vi "Logging Message Loop_temp.vi"(8 "error in (no error)":errorcluster, 10 "Data Queue":refnum<queue>, 11 "Message Queues":T1) -> (0 "error out":errorcluster)   [LabVIEW 2016]
doc: "The message loop subVI to handle messages pertaining to logging data."
uses:
  support/Message Queue/All Message Queues.ctl
  support/Message Queue/Message Cluster.ctl
  Logging Configuration.ctl
  Logging State.ctl
  support/Message Queue/Enqueue Message (Single).vi
  <vilib>/Utility/error.llb/Error Cluster From Error Code.vi
  <vilib>/ErrorRing/Error Ring.xnode
  Logging.lvlib
  support/Message Queue/Message Queue.lvlib
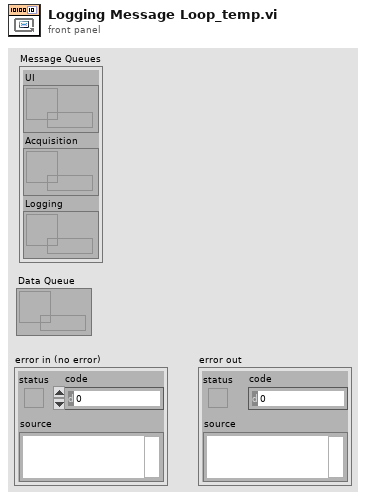
[diagram p1: front panel]
types:
  T1 = typedef "Message Queue.lvlib/All Message Queues.ctl" = cluster{"UI":refnum<queue>, "Acquisition":refnum<queue>, "Logging":refnum<queue>}
  T2 = typedef "Logging.lvlib/Logging State.ctl" = cluster{"State":enum16{"Logging", "Not Logging", "Idle"}, "Samples to Save":u32, "Force Trigger":bool}
  T3 = typedef "Logging.lvlib/Logging Configuration.ctl" = cluster{"Log File Base Path":path, "TDMS File Reference":refnum<k34>, "Samples to Save":u32, "Trigger - Time":u32, "Trigger - Threshold":dbl, "Trigger - Channel":u32, "Enable Time Trigger":bool, "Enable Threshold Trigger":bool, "Always Log":bool}
  T4 = enum16{"open", "open or create", "create or replace", "create", "open (read-only)"}
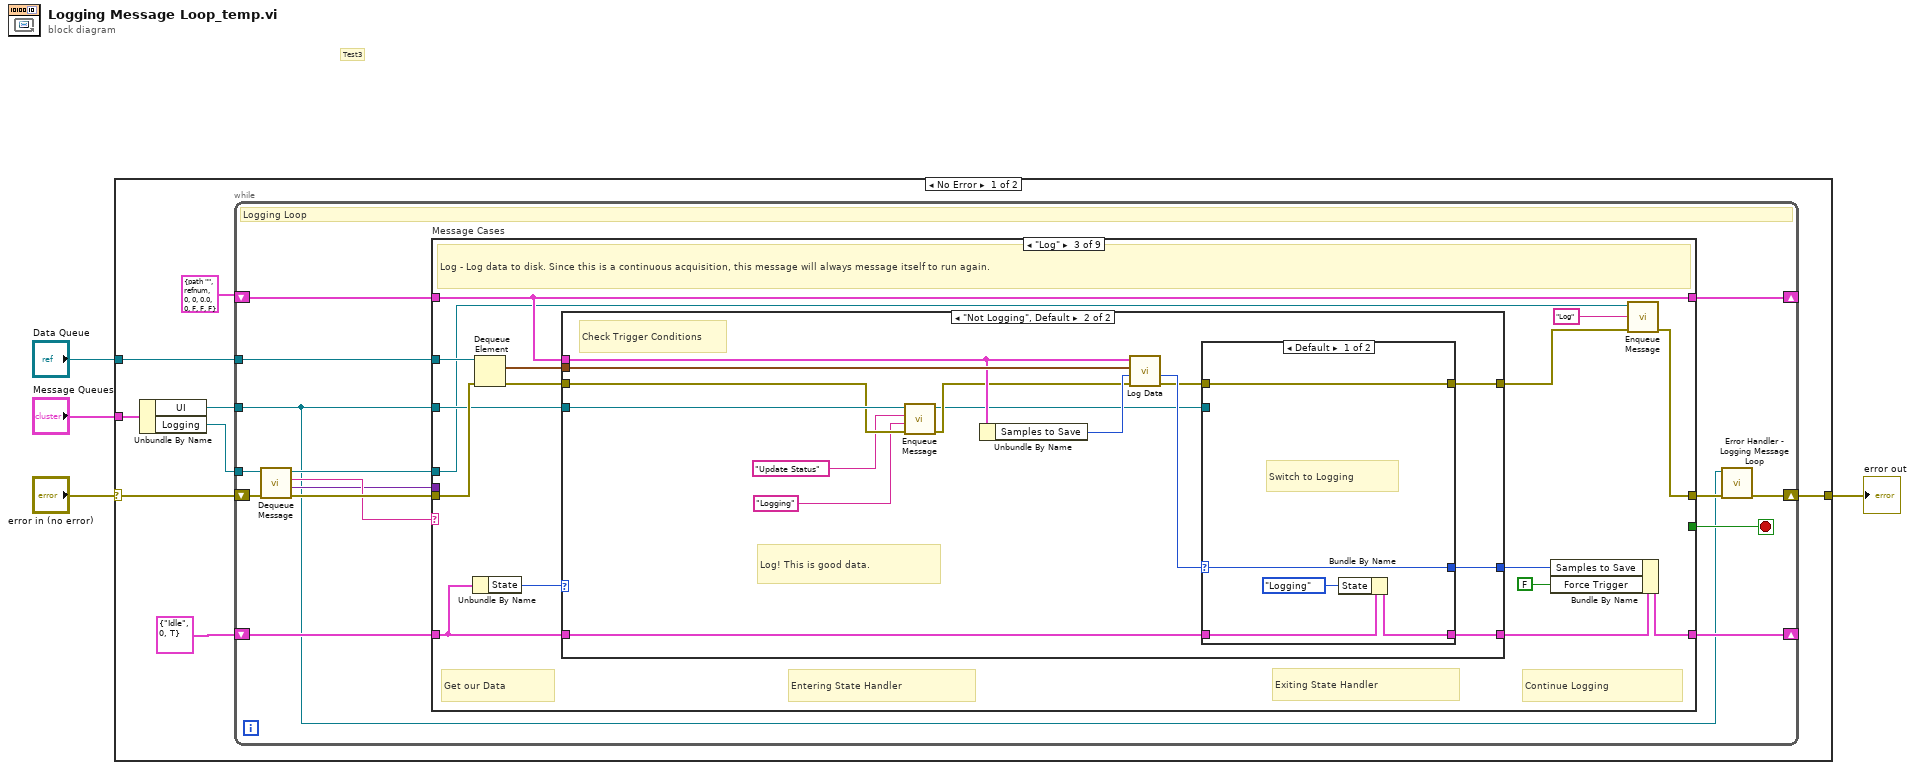
[diagram p0: block diagram]
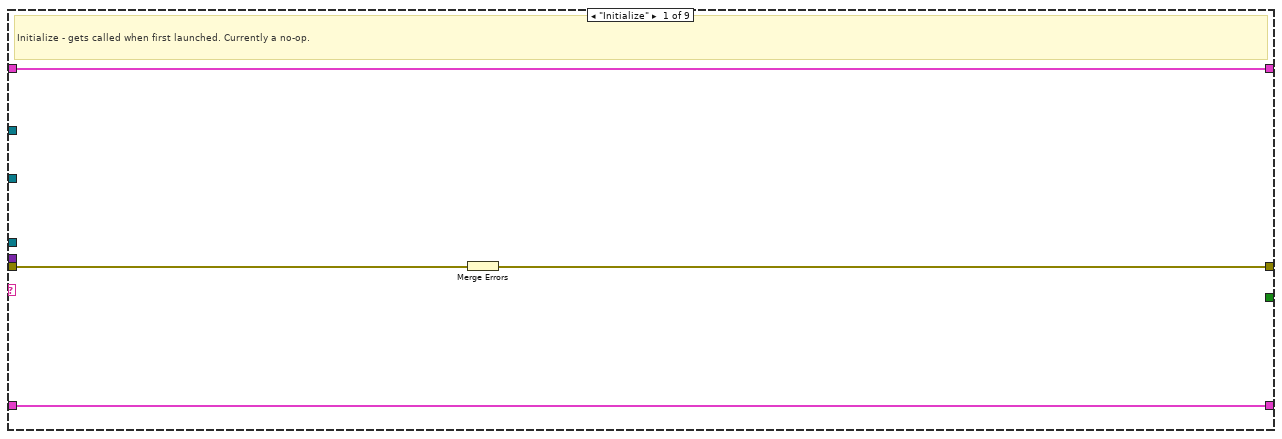
[diagram p2: hidden frame]
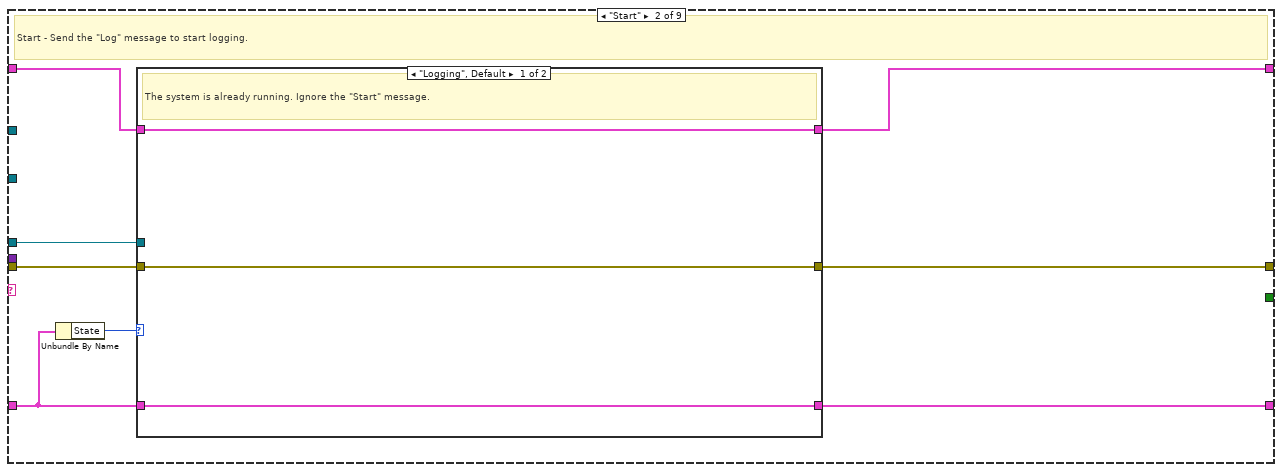
[diagram p3: hidden frame]
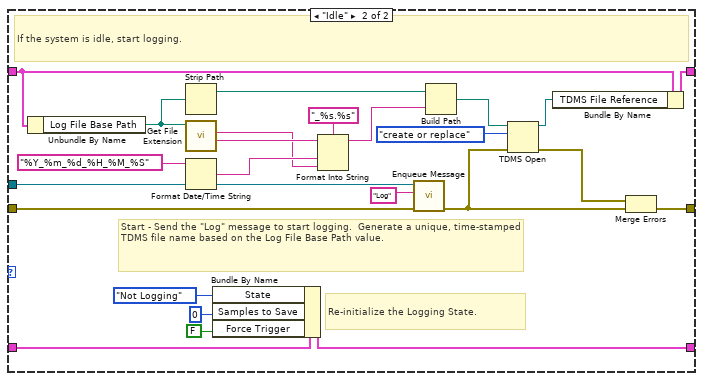
[diagram p4: hidden frame]
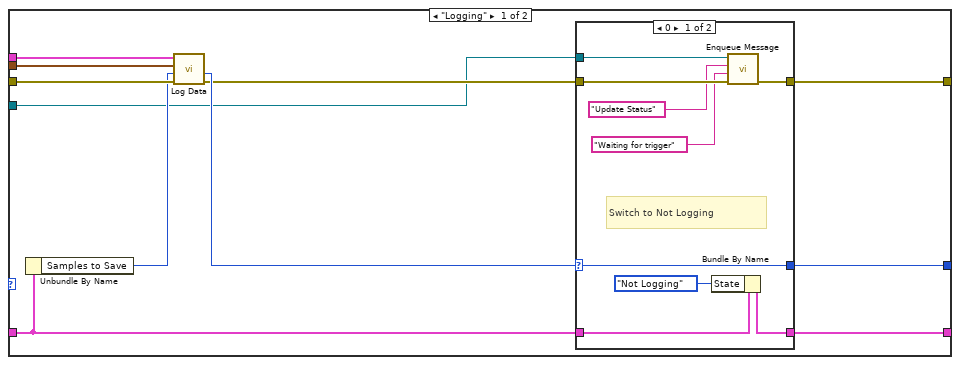
[diagram p5: hidden frame]
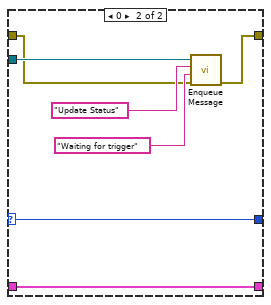
[diagram p7: hidden frame]
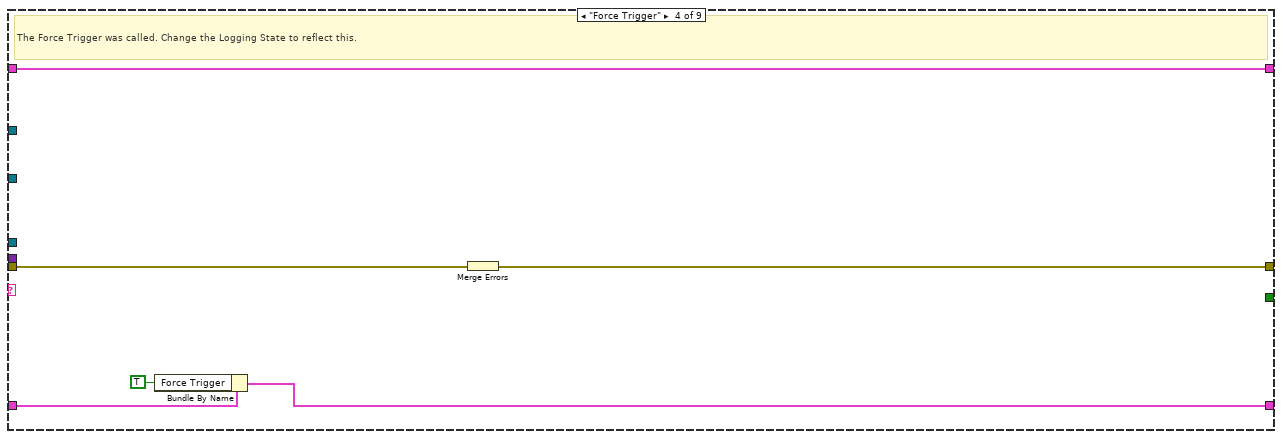
[diagram p8: hidden frame]
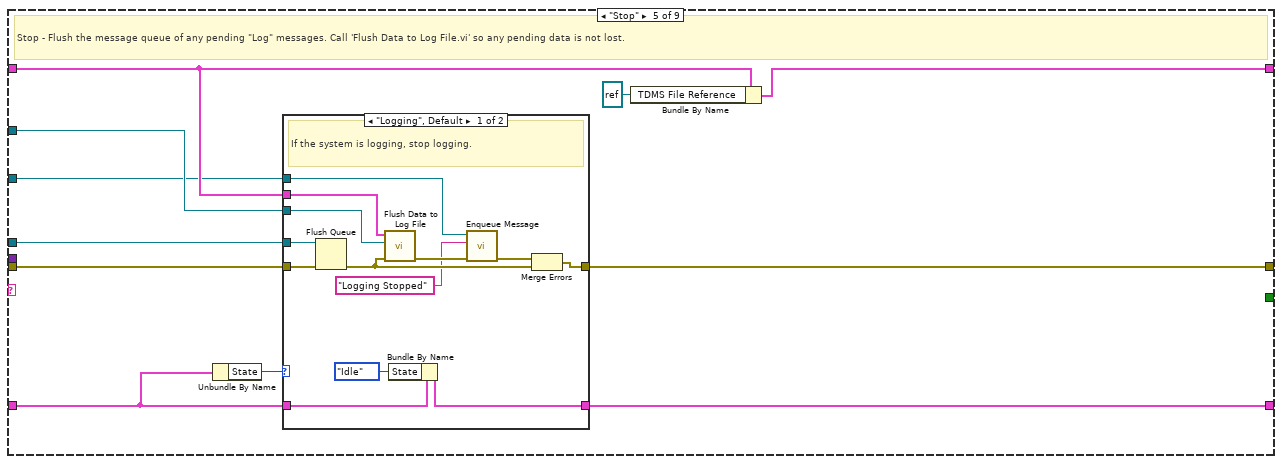
[diagram p9: hidden frame]
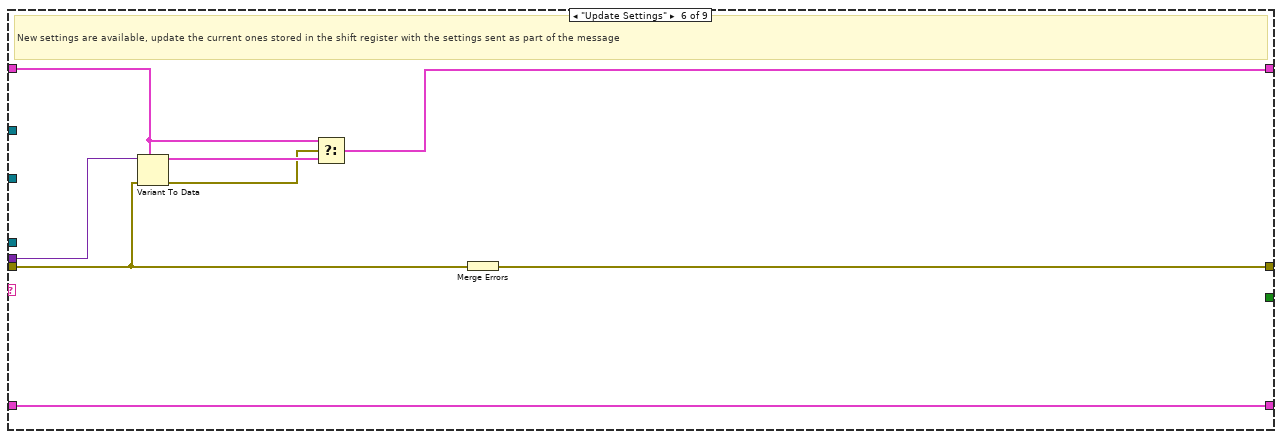
[diagram p11: hidden frame]
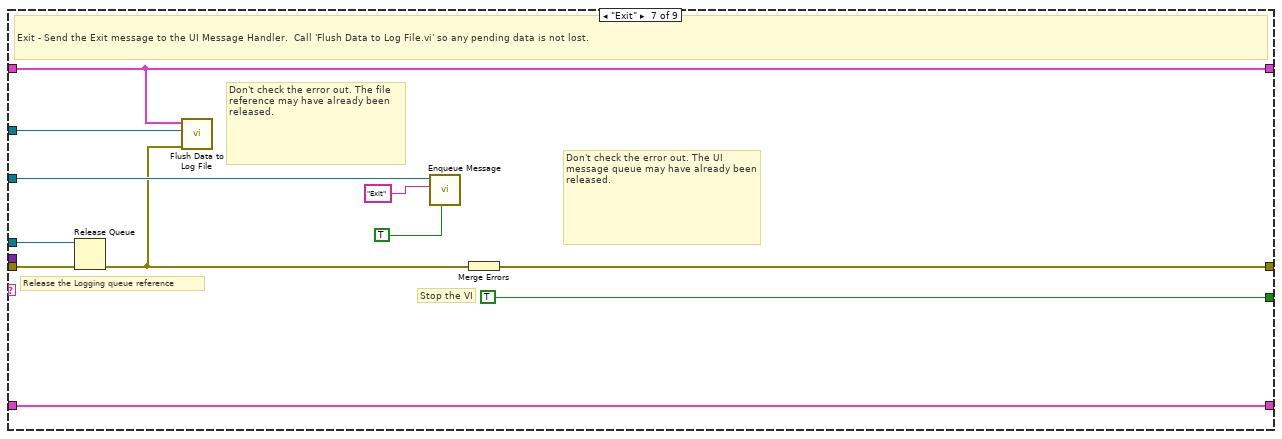
[diagram p12: hidden frame]
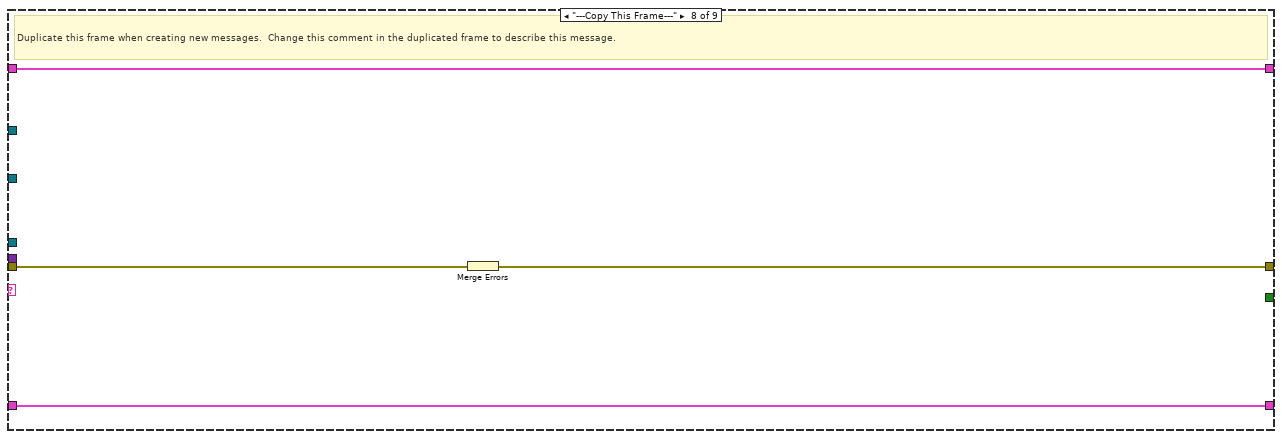
[diagram p13: hidden frame]
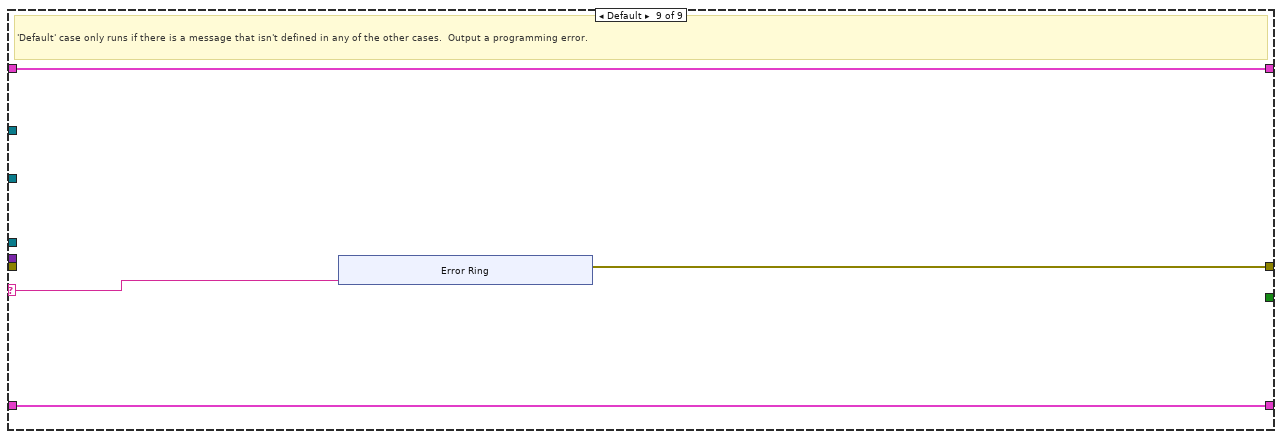
[diagram p14: hidden frame]
diagram:
  # "Test3"
  n1 = case shown="No Error" "error in (no error)" {
    selector: "error in (no error)" -> [w8 w199]
    tunnel: "Message Queues" -> [w12 _]
    tunnel: [w10 w199] -> w3
    tunnel: "Data Queue" -> [w7 _]
    frame No Error {
      n2 = Unbundle By Name(w12) -> ("UI"=w6:refnum<queue>, "Logging"=w11:refnum<queue>)
      n3 = while {
        tunnel: w11 -> [w19]
        shift-right: [w26] -> _
        shift-left: T3 {"Log File Base Path"=path "", "TDMS File Reference"=refnum, "Samples to Save"=0, "Trigger - Time"=0, "Trigger - Threshold"=0.0, "Trigger - Channel"=0, "Enable Time Trigger"=FALSE, "Enable Threshold Trigger"=FALSE, "Always Log"=FALSE} ("Logging Configuration") -> [w27]
        shift-right: [w14] -> w10
        shift-left: w8 -> [w24]
        tunnel: w6 -> [w13]
        tunnel: w7 -> [w18]
        shift-right: [w16] -> _
        shift-left: T2 {"State"=enum."Idle", "Samples to Save"=0, "Force Trigger"=TRUE} -> [w17]
        stop <- w25 stop-if-true
        # "Logging Loop"
        n4 = call "Dequeue Message.vi"("error in (no error)"=w24, "Message Queue"=w19) -> ("error out"=w23:errorcluster, "Message Data"=w21:variant, "Message"=w22:string, "dup Message Queue"=w20:refnum<queue>)  [unwired: 6 in]
        n5 = case "Message Cases" shown="\"Log\"" w22 {
          selector: w22 -> [_ _ _ _ _ _ _ _ w188]
          tunnel: w20 -> [_ w38 w70 _ w147 _ w177 _ _]
          tunnel: w23 -> [w29 w37 w80 w138 w148 w166 w180 w187 _]
          tunnel: [w31 w39 w82 w136 w149 w172 w182 w185 w189] -> w15
          tunnel: w27 -> [w30 w36 w75 w137 w144 w170 w176 w186 w191]
          tunnel: [w30 w35 w75 w137 w146 w167 w176 w186 w191] -> w26
          tunnel: [_ _ _ _ _ _ TRUE _ _] -> w25
          tunnel: w21 -> [_ _ _ _ _ w171 _ _ _]
          tunnel: w13 -> [_ _ w74 _ w142 _ w181 _ _]
          tunnel: w18 -> [_ _ w71 _ w143 _ w175 _ _]
          tunnel: w17 -> [w28 w33 w78 w135 w140 w165 w173 w184 w190]
          tunnel: [w28 w34 w73 w134 w139 w165 w173 w184 w190] -> w16
          frame "Initialize" {
            # "Initialize - gets called when first launched. Currently a no-op."
            n6 = Merge Errors(w29) -> (w31:errorcluster)
          }
          frame "Start" {
            # "Start - Send the \"Log\" message to start logging."
            n7 = Unbundle By Name(w33) -> ("State"=w32:enum16{"Logging", "Not Logging", "Idle"})
            n8 = case shown="\"Logging\", Default" w32 {
              tunnel: [w41 w66] -> w39
              tunnel: w38 -> [_ w65]
              tunnel: w37 -> [w41 w63]
              tunnel: w36 -> [w42 w54]
              tunnel: [w42 w51] -> w35
              tunnel: w33 -> [w40 w47]
              tunnel: [w40 w46] -> w34
              frame "Logging", Default {
                # "The system is already running. Ignore the \"Start\" message."
              }
              frame "Idle" {
                # "Re-initialize the Logging State."
                # "Start - Send the \"Log\" message to start logging.  Generate a unique, time-stamped TDMS file name based on the Log File Base Path value."
                # "If the system is idle, start logging."
                n9 = Unbundle By Name(w54) -> ("Log File Base Path"=w61:path)
                n10 = Strip Path(path=w61) -> (stripped path=w60:path)  [unwired: 1 out]
                n11 = call <vilib>:"Get File Extension.vi"("file"=w61) -> ("filename without extension"=w59:string, "lowercase file extension"=w56:string)  [unwired: 6 in, 3 out]
                n12 = Format Date/Time String(time format string (%c)="%Y_%m_%d_%H_%M_%S") -> (date/time string=w57:string)  [unwired: 2 in]
                n13 = Bundle By Name(cluster=w47, "State"=enum16{"Logging", "Not Logging"}."Not Logging", "Samples to Save"=u32 0 ("Reads to Save"), "Force Trigger"=FALSE) -> (w46:T2)
                n14 = Format Into String(format string="_%s.%s", initial string=w59, w57, w56) -> (resulting string=w55:string)  [unwired: 1 in, 1 out]
                n15 = call-poly "Enqueue Message.vi"("error in (no error)"=w63, "Message"="Log", "Message Queue"=w65) -> ("error out"=w49:errorcluster)  [unwired: 7 in, 1 out]
                n16 = Build Path(base path=w60, name or relative path=w55) -> (appended path=w52:path)
                n17 = TDMS Open(8:w49, 10:T4."create or replace" ("operation (0:open)"), 11:w52) -> (0:w48:errorcluster, 3:w53:refnum<k34>)  [unwired: 4 in]
                n18 = Bundle By Name(cluster=w54, "TDMS File Reference"=w53) -> (w51:T3)
                n19 = Merge Errors(w48, w49) -> (w66:errorcluster)
              }
            }
          }
          frame "Log" {
            # "Exiting State Handler"
            # "Continue Logging"
            # "Entering State Handler"
            # "Get our Data"
            # "Log - Log data to disk. Since this is a continuous acquisition, this message will always message itself to run again."
            n20 = Unbundle By Name(w78) -> ("State"=w79:enum16{"Logging", "Not Logging", "Idle"})
            n21 = Dequeue Element(queue=w71, error in (no error)=w80) -> (element=w77:waveform(dbl)[], error out=w76:errorcluster)  [unwired: 1 in, 2 out]
            n22 = case shown="\"Not Logging\", Default" w79 {
              tunnel: [w87 w120] -> w69
              tunnel: w78 -> [w88 w118]
              tunnel: w77 -> [w92 w114]
              tunnel: w76 -> [w91 w115]
              tunnel: w75 -> [w93 w113]
              tunnel: w74 -> [w83 w117]
              tunnel: [w84 w119] -> w67
              tunnel: [w86 w116] -> w68
              frame "Logging" {
                n23 = Unbundle By Name(w88) -> ("Samples to Save"=w90:u32)
                n24 = call "Log Data.vi"("error in (no error)"=w91, "Samples to Save In"=w90, "Data"=w92, "Logging Configuration"=w93) -> ("error out"=w85:errorcluster, "Samples to Save Out"=w89:u32)  [unwired: 6 in]
                n25 = case shown="0" w89 {
                  selector: w89 -> [w99 w105]
                  tunnel: w85 -> [w97 w104]
                  tunnel: [w98 w104] -> w84
                  tunnel: w88 -> [w101 w103]
                  tunnel: [w100 w103] -> w87
                  tunnel: [w99 w105] -> w86
                  tunnel: w83 -> [w94 _]
                  frame 0 {
                    # "Switch to Not Logging"
                    n26 = Bundle By Name(cluster=w101, "State"=enum16{"Logging", "Not Logging"}."Not Logging") -> (w100:T2)
                    n27 = call-poly "Enqueue Message.vi"("error in (no error)"=w97, "Message Data"="Waiting for trigger" ("Waiting for trigger"), "Message"="Update Status", "Message Queue"=w94) -> ("error out"=w98:errorcluster)  [unwired: 6 in, 1 out]
                  }
                  frame Default {
                    # "Continue in our same State."
                  }
                }
              }
              frame "Not Logging", Default {
                # "Log! This is good data."
                # "Check Trigger Conditions"
                n28 = call-poly "Enqueue Message.vi"("error in (no error)"=w115, "Message Data"="Logging" ("Logging"), "Message"="Update Status", "Message Queue"=w117) -> ("error out"=w109:errorcluster, "dup Message Queue"=w106:refnum<queue>)  [unwired: 6 in]
                n29 = Unbundle By Name(w113) -> ("Samples to Save"=w110:u32)
                n30 = call "Log Data.vi"("error in (no error)"=w109, "Samples to Save In"=w110, "Data"=w114, "Logging Configuration"=w113) -> ("error out"=w107:errorcluster, "Samples to Save Out"=w108:u32)  [unwired: 6 in]
                n31 = case shown="Default" w108 {
                  selector: w108 -> [w125 w132]
                  tunnel: [w125 w132] -> w116
                  tunnel: [w122 w131] -> w120
                  tunnel: w118 -> [w123 w131]
                  tunnel: w107 -> [w121 w127]
                  tunnel: [w121 w126] -> w119
                  tunnel: w106 -> [_ w130]
                  frame Default {
                    # "Switch to Logging"
                    n32 = Bundle By Name(cluster=w123, "State"=enum16{"Logging", "Not Logging"}."Logging") -> (w122:T2)
                  }
                  frame 0 {
                    n33 = call-poly "Enqueue Message.vi"("error in (no error)"=w127, "Message Data"="Waiting for trigger" ("Waiting for trigger"), "Message"="Update Status", "Message Queue"=w130) -> ("error out"=w126:errorcluster)  [unwired: 6 in, 1 out]
                  }
                }
              }
            }
            n34 = Bundle By Name(cluster=w69, "Samples to Save"=w68, "Force Trigger"=FALSE) -> (w73:T2)
            n35 = call-poly "Enqueue Message.vi"("error in (no error)"=w67, "Message"="Log", "Message Queue"=w70) -> ("error out"=w82:errorcluster)  [unwired: 7 in, 1 out]
          }
          frame "Force Trigger" {
            # "The Force Trigger was called. Change the Logging State to reflect this."
            n36 = Bundle By Name(cluster=w135, "Force Trigger"=TRUE) -> (w134:T2)
            n37 = Merge Errors(w138) -> (w136:errorcluster)
          }
          frame "Stop" {
            # "Stop - Flush the message queue of any pending \"Log\" messages. Call 'Flush Data to Log File.vi' so any pending data is not lost."
            n38 = Unbundle By Name(w140) -> ("State"=w141:enum16{"Logging", "Not Logging", "Idle"})
            n39 = case shown="\"Logging\", Default" w141 {
              tunnel: [w162 w164] -> w149
              tunnel: w148 -> [w161 w164]
              tunnel: w147 -> [w160 _]
              tunnel: w144 -> [w159 _]
              tunnel: w143 -> [w158 _]
              tunnel: w142 -> [w154 _]
              tunnel: w140 -> [w152 w163]
              tunnel: [w151 w163] -> w139
              frame "Logging", Default {
                # "If the system is logging, stop logging."
                n40 = Flush Queue(queue=w160, error in (no error)=w161) -> (error out=w157:errorcluster)  [unwired: 2 out]
                n41 = call "Flush Data to Log File.vi"("error in (no error)"=w157, "Data Queue"=w158, "Logging Configuration"=w159) -> ("error out"=w156:errorcluster)  [unwired: 8 in]
                n42 = Bundle By Name(cluster=w152, "State"=enum16{"Logging", "Not Logging", "Idle"}."Idle") -> (w151:T2)
                n43 = call-poly "Enqueue Message.vi"("error in (no error)"=w156, "Message"="Logging Stopped", "Message Queue"=w154) -> ("error out"=w155:errorcluster)  [unwired: 7 in, 1 out]
                n44 = Merge Errors(w155, w157) -> (w162:errorcluster)
              }
              frame "Idle" {
                # "The system is already idle. Ignore the \"Stop\" message."
              }
            }
            n45 = Bundle By Name(cluster=w144, "TDMS File Reference"=refnum<k34> refnum ("tdms file out")) -> (w146:T3)
          }
          frame "Update Settings" {
            # "New settings are available, update the current ones stored in the shift register with the settings sent as part of the message"
            n46 = Variant To Data(error in=w166, type=w170, Variant=w171) -> (data=w169:T3, error out=w168:errorcluster)
            n47 = Select(t=w170, s=w168, f=w169) -> (s? t:f=w167:T3)
            n48 = Merge Errors(w166) -> (w172:errorcluster)
          }
          frame "Exit" {
            # "Don't check the error out. The file reference may have already been released."
            # "Release the Logging queue reference"
            # "Don't check the error out. The UI message queue may have already been released."
            # "Stop the VI"
            # "Exit - Send the Exit message to the UI Message Handler.  Call 'Flush Data to Log File.vi' so any pending data is not lost."
            n49 = Release Queue(queue=w177, error in (no error)=w180) -> (error out=w174:errorcluster)  [unwired: 1 in, 2 out]
            n50 = call "Flush Data to Log File.vi"("error in (no error)"=w174, "Data Queue"=w175, "Logging Configuration"=w176) -> ()  [unwired: 8 in, 1 out]
            n51 = call-poly "Enqueue Message.vi"("Priority Message? (F)"=TRUE, "Message"="Exit", "Message Queue"=w181) -> ()  [unwired: 7 in, 2 out]
            n52 = Merge Errors(w174) -> (w182:errorcluster)
          }
          frame "---Copy This Frame---" {
            # "Duplicate this frame when creating new messages.  Change this comment in the duplicated frame to describe this message."
            n53 = Merge Errors(w187) -> (w185:errorcluster)
          }
          frame Default {
            # "'Default' case only runs if there is a message that isn't defined in any of the other cases.  Output a programming error."
            n54 = xnode "Error Ring"("parameter 0"=w188) -> ("error out"=w189:errorcluster)
          }
        }
        n55 = call "Error Handler - Logging Message Loop.vi"("error in (no error)"=w15, "Message Queue"=w13) -> ("dup error in"=w14:errorcluster)  [unwired: 8 in, 1 out]
      }
    }
    frame Error {
    }
  }
  "error out" <- w3
